vi "Ok Prompt If Error.vi"(8 "error in":errorcluster, 11 "Message":string) -> (0 "error out":errorcluster)   [LabVIEW 2018]
panel:
  in  "OK Button":bool
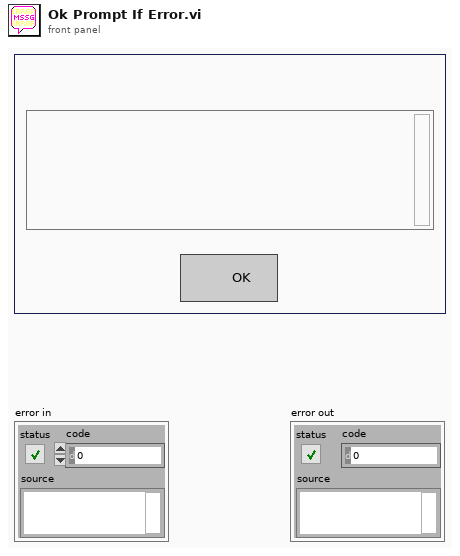
[diagram p1: front panel]
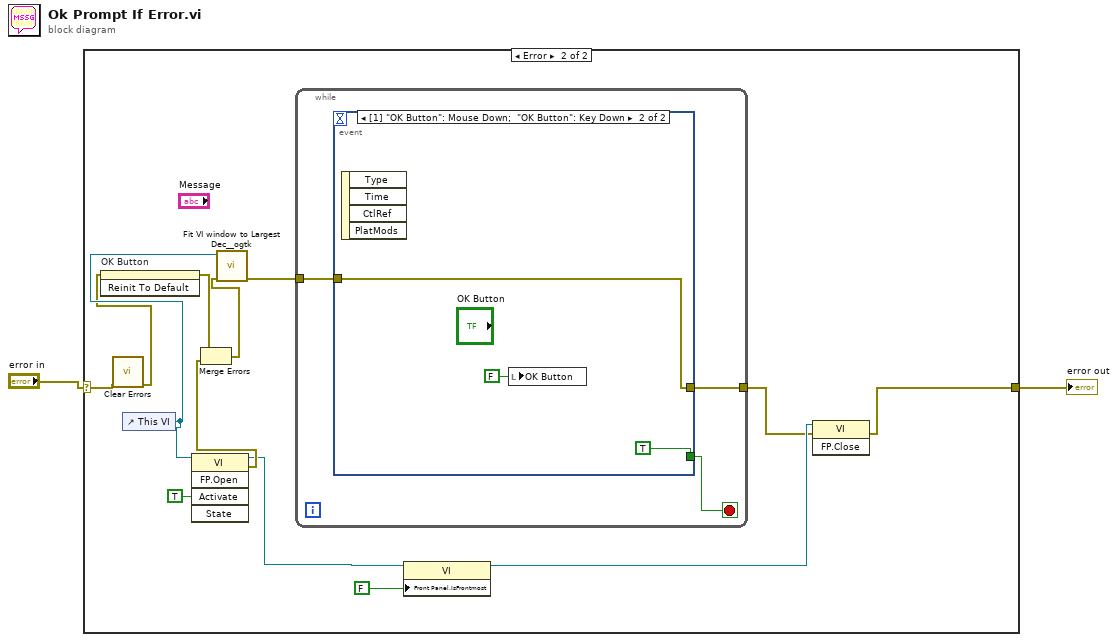
[diagram p0: block diagram]
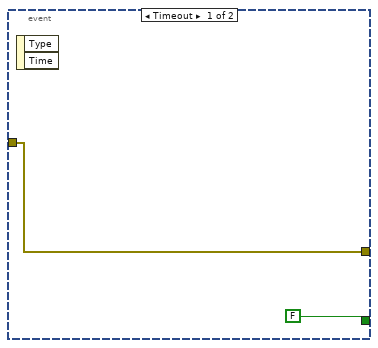
[diagram p3: hidden frame]
diagram:
  n1 = case shown="Error" "error in" {
    selector: "error in" -> [w3 w7]
    tunnel: [w3 w8] -> w1
    frame No Error {
    }
    frame Error {
      n2 = call <vilib>:"Clear Errors.vi"("error in (no error)"=w7) -> ("error out"=w6:errorcluster)  [unwired: 5 in, 1 out]
      n3 = invoke on="OK Button" class="Bool (strict)" method="Reinit To Default"(error in=w6) -> (error out=w14:errorcluster)  [unwired: 2 in, 2 out]
      n4 = control-ref of="This VI"() -> (w11:refnum<vi>)
      n5 = invoke class="VI" method="FP.Open"(reference=w11, "Activate"=TRUE ("Activate?")) -> (reference out=w5:refnum<vi>, error out=w12:errorcluster)  [unwired: 3 in, 3 out]
      n6 = Merge Errors(w14, w12) -> (w13:errorcluster)
      n7 = call <userlib>:"Fit VI window to Largest Dec__ogtk.vi"("error in (no error)"=w13, "VI Ref (calling VI)"=w11) -> ("error out"=w15:errorcluster)  [unwired: 4 in, 1 out]
      n8 = while {
        tunnel: w15 -> [w19]
        tunnel: [w18] -> w9
        stop <- w17 stop-if-true
        n9 = event shown="[1] \"OK Button\": Mouse Down;  \"OK Button\": Key Down" {
          selector: _ -> [_ _]
          dyn-events: _ -> [_ _]
          timeout: _ -> [_ _]
          tunnel: w19 -> [w21 w22]
          tunnel: [w21 w22] -> w18
          tunnel: [FALSE TRUE] -> w17
          event Timeout {
            n10 = event-data() -> ()  [unwired: 1 in, 2 out]
          }
          event "OK Button": Mouse Down; "OK Button": Key Down {
            n11 = event-data() -> ()  [unwired: 1 in, 4 out]
            n12 = local write "OK Button"(FALSE ("OK Button")) -> ()
          }
        }
      }
      n13 = property class="VI"(reference=w5, "Front Panel.IsFrontmost"=FALSE ("Front Panel Window:Is Frontmost")) -> (reference out=w10:refnum<vi>)  [unwired: 1 in, 1 out]
      n14 = invoke class="VI" method="FP.Close"(reference=w10, error in=w9) -> (error out=w8:errorcluster)  [unwired: 1 in, 2 out]
    }
  }
  "error out" <- w1
